vi "LWXPS_RequestType1.vi"(0 "XPS Reference IN":refnum<k24>, 7 "LabVIEW error IN":errorcluster) -> (10 "XPS Reference OUT":refnum<k24>, 11 "LabVIEW error OUT":errorcluster, 12 "Returned error code":i32, 13 "XPS Error String":string, 14 "Header":string, 15 "Y Sin Cos":string, 16 "Time Stamp":string, 17 "X Sin Cos":string, 18 "1 D Fe":string, 19 "Y Motor":string, 20 "1 D Position":string, 21 "X Fe":string, 22 "X Position":string, 23 "Yaw Fe":string, 24 "Yaw Position":string, 25 "Y Fe":string, 26 "Y Position":string, 27 "X Motor":string)   [LabVIEW 2014]
uses:
  D:/XPSQ8_LabView_Library/Development/Source/Dll/Newport.XPS.CommandInterface.dll
  Dll/Newport.XPS.CommandInterface.dll
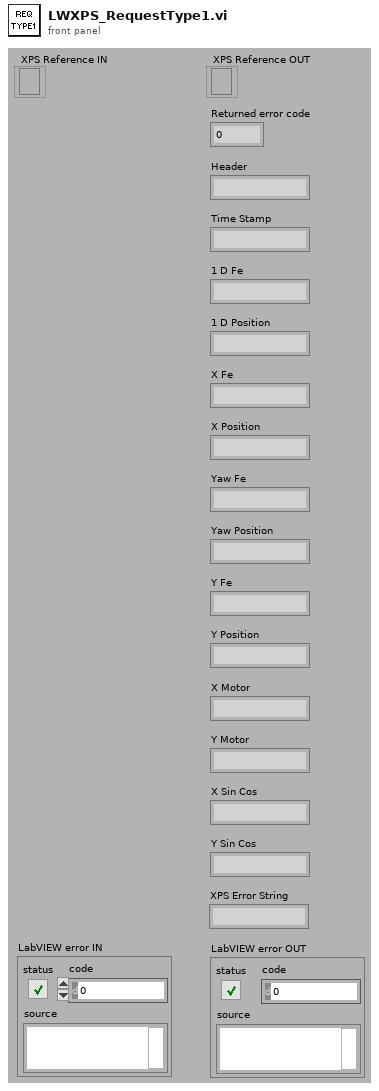
[diagram p1: front panel]
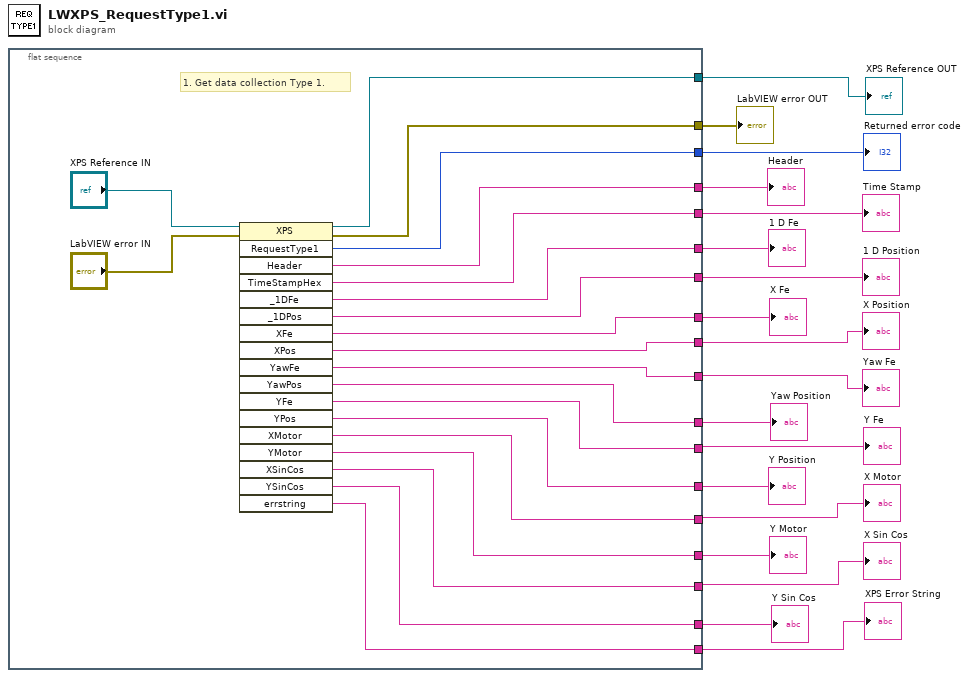
[diagram p0: block diagram]
diagram:
  n1 = flat-sequence {
    tunnel: [w37] -> w18
    tunnel: [w35] -> w17
    tunnel: [w30] -> w16
    tunnel: [w34] -> w15
    tunnel: [w33] -> w13
    tunnel: [w32] -> w11
    tunnel: [w31] -> w14
    tunnel: [w29] -> w12
    tunnel: [w28] -> w10
    tunnel: [w27] -> w9
    tunnel: [w26] -> w8
    tunnel: [w25] -> w7
    tunnel: [w24] -> w6
    tunnel: [w23] -> w5
    tunnel: [w22] -> w4
    tunnel: [w21] -> w3
    tunnel: [w20] -> w2
    tunnel: [w19] -> w1
    frame #0 {
      # "1. Get data collection Type 1."
      n2 = invoke class="XPS" method="RequestType1"(reference="XPS Reference IN", error in="LabVIEW error IN") -> (reference out=w37:refnum<k24>, error out=w35:errorcluster, "RequestType1"=w30:i32, "Header"=w31:string, "TimeStampHex"=w34:string, "_1DFe"=w33:string, "_1DPos"=w32:string, "XFe"=w29:string, "XPos"=w28:string, "YawFe"=w27:string, "YawPos"=w26:string, "YFe"=w25:string, "YPos"=w24:string, "XMotor"=w23:string, "YMotor"=w22:string, "XSinCos"=w21:string, "YSinCos"=w20:string, "errstring"=w19:string)  [unwired: 16 in]
    }
  }
  "X Fe" <- w12
  "XPS Reference OUT" <- w18
  "LabVIEW error OUT" <- w17
  "Returned error code" <- w16
  "Time Stamp" <- w15
  "Header" <- w14
  "1 D Fe" <- w13
  "1 D Position" <- w11
  "X Position" <- w10
  "Yaw Fe" <- w9
  "Yaw Position" <- w8
  "Y Fe" <- w7
  "Y Position" <- w6
  "X Motor" <- w5
  "Y Motor" <- w4
  "X Sin Cos" <- w3
  "Y Sin Cos" <- w2
  "XPS Error String" <- w1
